vi "manage comm restablished.vi"(8 "error in (no error)":errorcluster, 11 "Channel in":refnum<class "SPARC4_Channel.lvclass">) -> (0 "error out":errorcluster, 3 "Channel out":refnum<class "SPARC4_Channel.lvclass">)   [LabVIEW 2018, in "SPARC4_Channel.lvclass"]
uses:
  SPARC4_Channel.lvclass
  Server/Server.lvclass
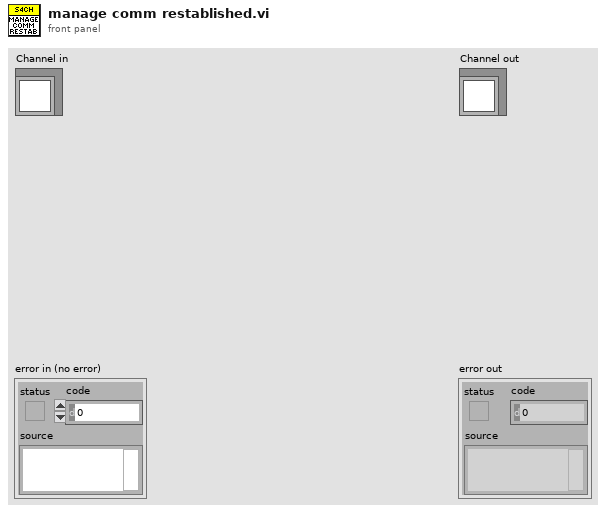
[diagram p1: front panel]
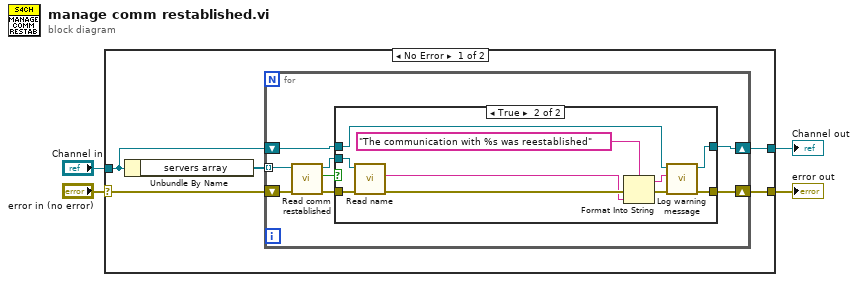
[diagram p0: block diagram]
diagram:
  n1 = case shown="No Error" "error in (no error)" {
    selector: "error in (no error)" -> [w8 w31]
    tunnel: [w7 w31] -> w1
    tunnel: [w6 w30] -> w2
    tunnel: "Channel in" -> [w9 w30]
    frame No Error {
      n2 = Unbundle By Name(w9) -> ("servers array"=w5:refnum<class "Server.lvclass">[])
      n3 = for {
        shift-right: [w16] -> w6
        shift-left: w9 -> [w17]
        shift-right: [w15] -> w7
        shift-left: w8 -> [w14]
        tunnel: w5 -> [w11] mode=indexing
        n4 = call-dynamic "Read comm restablished.vi"("error in (no error)"=w14, "Server in"=w11) -> ("error out"=w10:errorcluster, "comm restablished"=w13:bool, "Server out"=w12:refnum<class "Server.lvclass">)  [unwired: 7 in]
        n5 = case shown="True" w13 {
          tunnel: w17 -> [w19 w21]
          tunnel: [w19 w20] -> w16
          tunnel: [w18 w22] -> w15
          tunnel: w12 -> [_ w28]
          tunnel: w10 -> [w18 w26]
          frame False {
          }
          frame True {
            n6 = call-dynamic "Read name.vi"("error in (no error)"=w26, "Server in"=w28) -> ("error out"=w27:errorcluster, "name"=w25:string)  [unwired: 7 in, 1 out]
            n7 = Format Into String(format string="The communication with %s was reestablished", error in=w27, w25) -> (resulting string=w24:string, error out=w23:errorcluster)  [unwired: 1 in]
            n8 = call "Log warning message.vi"("error in (no error)"=w23, "String"=w24, "Channel in"=w21) -> ("error out"=w22:errorcluster, "Channel out"=w20:refnum<class "SPARC4_Channel.lvclass">)  [unwired: 7 in]
          }
        }
      }
    }
    frame Error {
    }
  }
  "error out" <- w1
  "Channel out" <- w2
